vi "nhap-baocao.vi"() -> ()   [LabVIEW 2015]
uses:
  Report (lvlib)/Report - CSV/Report - CSV.lvlib
panel:
  out "Quantity":string
  out "Mass":string
  out "ID":string
  out "C/N":string="b6783\nQuantity: 35\nMass: 2.94"
  out "DATA":string
  in  "delete":bool
  in  "File name .csv":string
  out "STT":dbl format="%#_13g"
  in  "stop":bool
  in  "Boolean":bool
  in  "Path save data report":path=path "C:/Data"
  in  "Result":i32(listbox)
  # "Table Result"
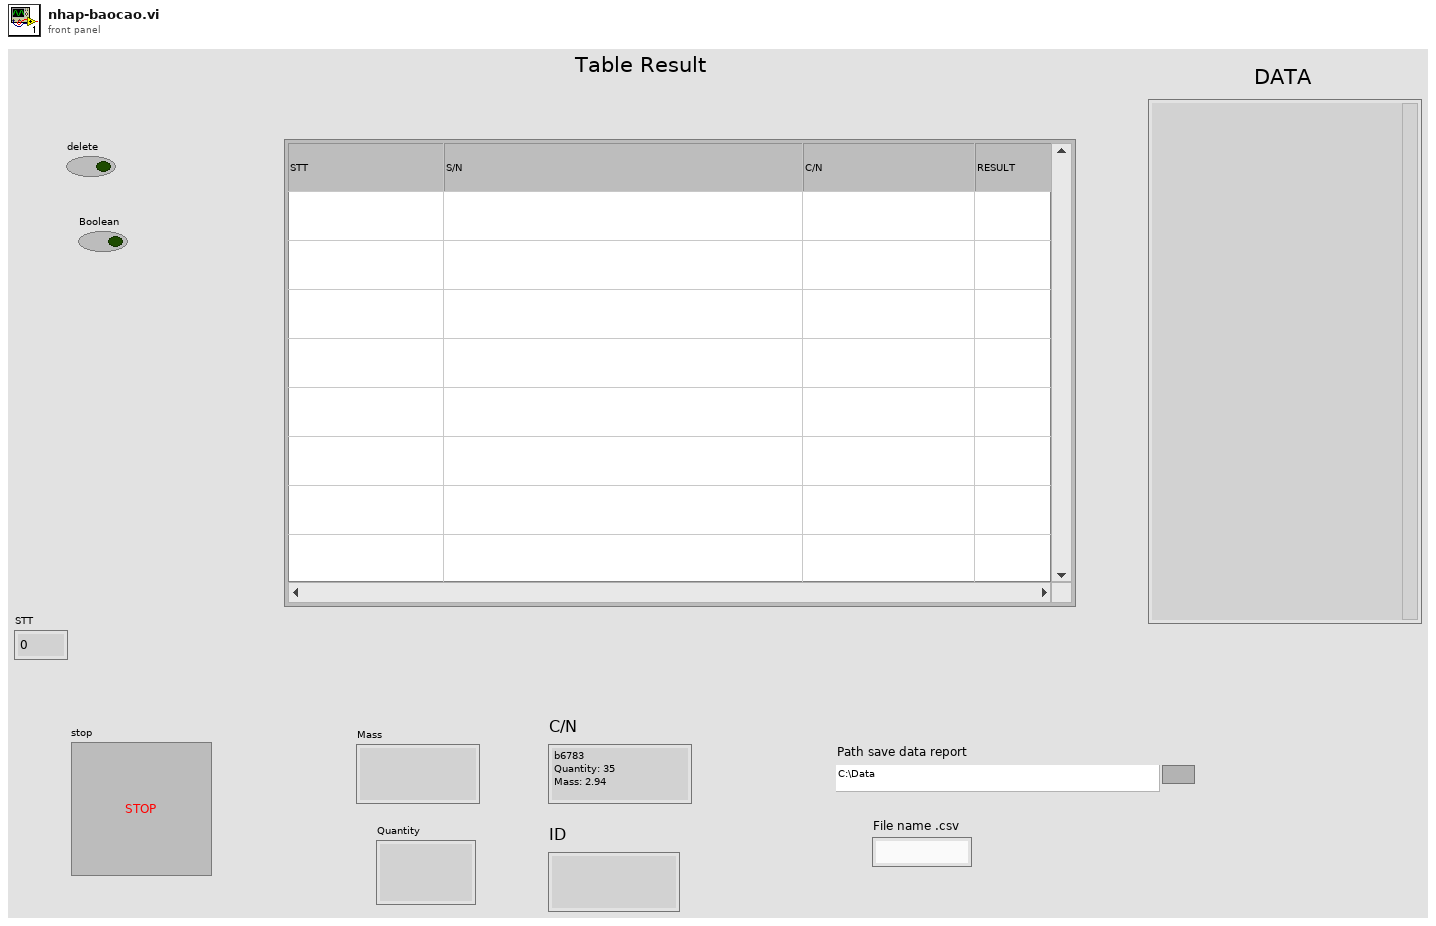
[diagram p1: front panel]
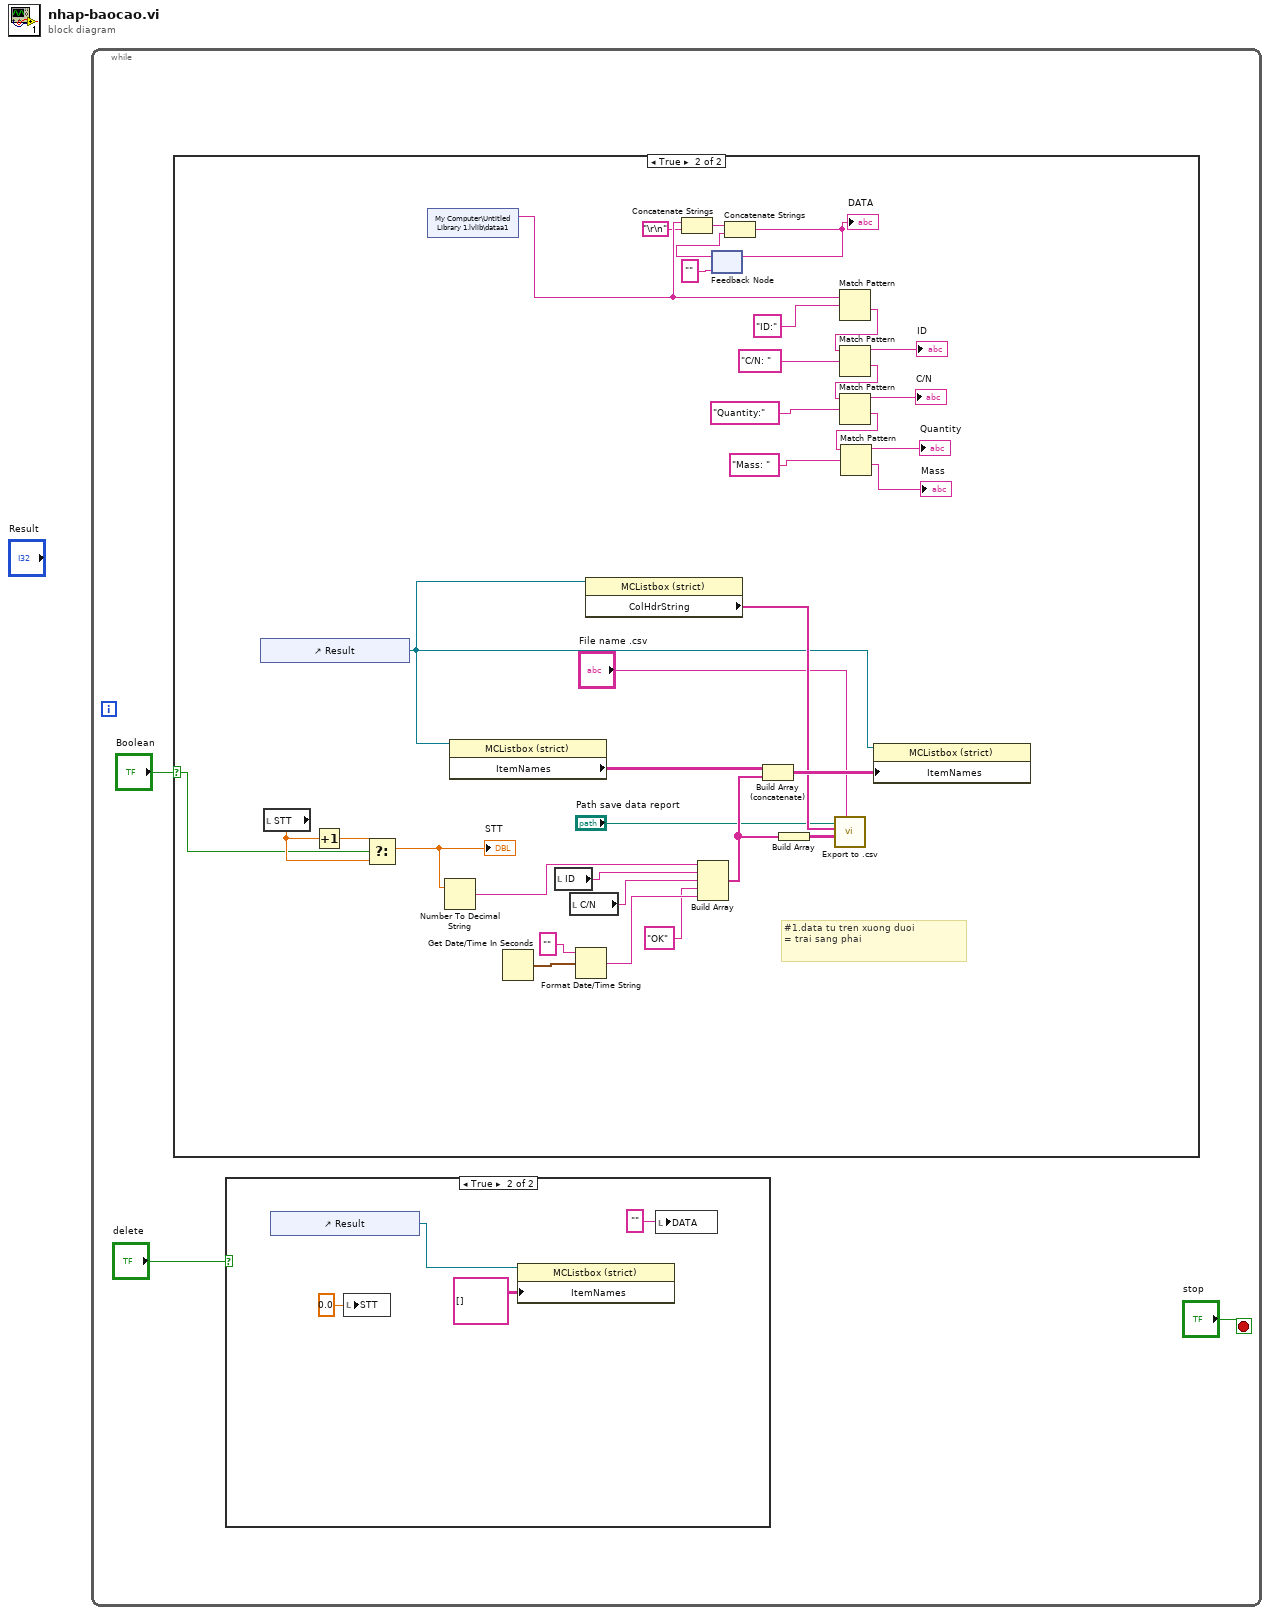
[diagram p0: block diagram]
diagram:
  n1 = while {
    stop <- "stop" stop-if-true
    n2 = case shown="True" "Boolean" {
      selector: "Boolean" -> [_ w33]
      frame False {
      }
      frame True {
        # "#1.data tu tren xuong duoi\n= trai sang phai"
        n3 = control-ref of="Result"() -> (w36:refnum<vi>)
        n4 = local read "STT"() -> (w35:dbl)
        n5 = Increment(x=w35) -> (x+1=w34:dbl)
        n6 = Select(t=w34, s=w33, f=w35) -> (s? t:f=w32:dbl)
        "STT" <- w32
        n7 = shared-variable "My Computer\\Untitled Library 1.lvlib\\dataa1"() -> (w28:string)  [unwired: 1 in, 1 out]
        n8 = Number To Decimal String(number=w32) -> (decimal integer string=w22:string)  [unwired: 1 in]
        n9 = property on="Property Node" class="MCListbox (strict)"(reference=w36) -> ("ItemNames"=w43:string[][])  [unwired: 1 in, 2 out]
        n10 = Get Date/Time In Seconds() -> (seconds since 1Jan1904=w41:timestamp)
        n11 = local read "ID"() -> (w9:string)
        n12 = local read "C/N"() -> (w8:string)
        n13 = Format Date/Time String(time format string (%c)="", seconds (now)=w41) -> (date/time string=w30:string)  [unwired: 1 in]
        n14 = property on="Property Node" class="MCListbox (strict)"(reference=w36) -> ("ColHdrString"=w38:string[])  [unwired: 1 in, 2 out]
        n15 = Concatenate Strings(w28, "\r\n" ("End of Line Constant")) -> (w25:string)
        n16 = Build Array(w22, w9, w8, "OK" ("element"), w30) -> (w40:string[])
        n17 = feedback #1("") -> (w24:string)
        n18 = Concatenate Strings(w25, w24) -> (w23:string)
        "DATA" <- w23
        n19 = feedback-in #1(w23) -> ()
        n20 = Build Array (concatenate)(w43, w40) -> (w42:string[][])
        n21 = Build Array(w40) -> (w39:string[][])
        n22 = call "Export to .csv"("File name .csv"="File name .csv", "Data - 2D"=w39, "ColHdrString - 1D"=w38, "Path in"="Path save data report") -> ()  [unwired: 8 in]
        n23 = Match Pattern(string=w28, regular expression="ID:") -> (after substring=w20:string)  [unwired: 1 in, 3 out]
        n24 = Match Pattern(string=w20, regular expression="C/N: ") -> (before substring=→"ID":string, after substring=w19:string)  [unwired: 1 in, 2 out]
        n25 = Match Pattern(string=w19, regular expression="Quantity:") -> (before substring=→"C/N":string, after substring=w14:string)  [unwired: 1 in, 2 out]
        n26 = Match Pattern(string=w14, regular expression="Mass: ") -> (before substring=→"Quantity":string, after substring=→"Mass":string)  [unwired: 1 in, 2 out]
        n27 = property on="Property Node" class="MCListbox (strict)"(reference=w36, "ItemNames"=w42) -> ()  [unwired: 1 in, 2 out]
      }
    }
    n28 = case shown="True" "delete" {
      frame False {
      }
      frame True {
        n29 = control-ref of="Result"() -> (w7:refnum<vi>)
        n30 = local write "STT"(0.0 ("STT")) -> ()
        n31 = property on="Property Node" class="MCListbox (strict)"(reference=w7, "ItemNames"=string[][] [] ("Item Names")) -> ()  [unwired: 1 in, 2 out]
        n32 = local write "DATA"("" ("DATA")) -> ()
      }
    }
  }
